vi "qWGI.vi"(0 "System no.":i32=1 min=1 max=4 step=1, 2 "Generator ID":string[](array[string]), 3 "All IDs?":bool, 4 "identifier?":bool=TRUE, 5 "error in":errorcluster) -> (14 "WGI parameter":i32[](array[numeric]), 19 "error out":errorcluster)   [LabVIEW 2026]
doc: "Returns the index of the currently output wave point.\n\nE-709: Generator ID can be 1. If All IDs? = TRUE, then identifier? must be FALSE."
panel:
  # "Returns the index of the currently output wave point"
  # "If all IDs: use"
  # "Query"
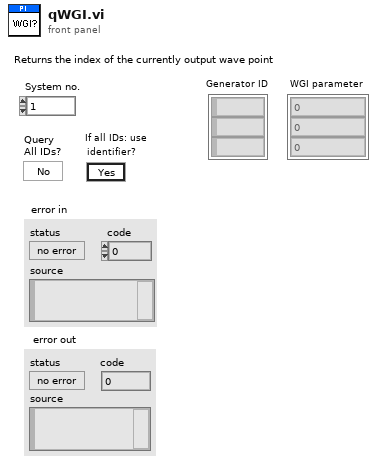
[diagram p1: front panel]
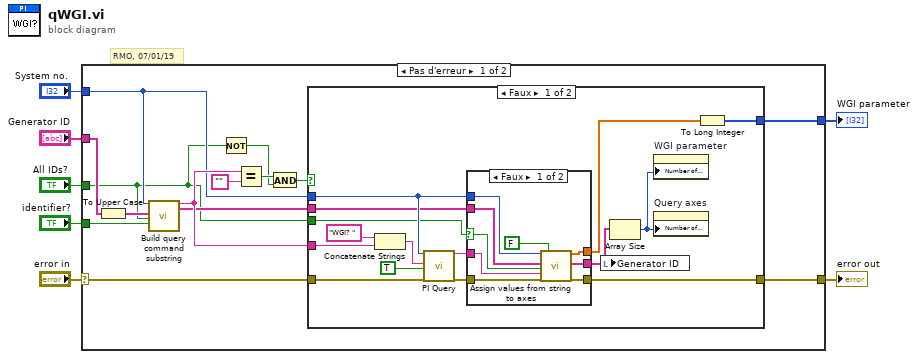
[diagram p0: block diagram]
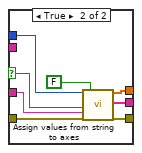
[diagram p2: hidden frame]
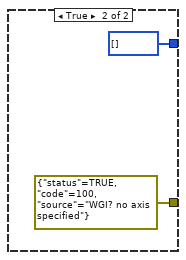
[diagram p3: hidden frame]
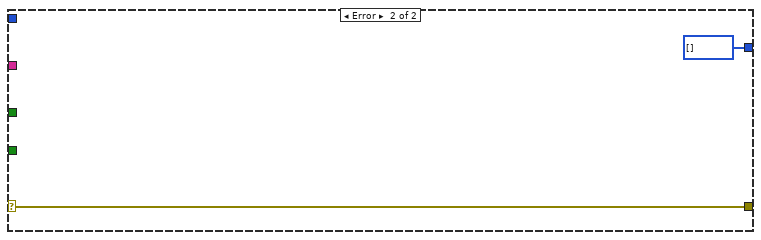
[diagram p4: hidden frame]
diagram:
  # "RMO, 07/01/19"
  n1 = case shown="Pas d'erreur" "error in" {
    selector: "error in" -> [w10 w57]
    tunnel: [w21 i32[] []] -> w7
    tunnel: "Generator ID" -> [w20 _]
    tunnel: [w8 w57] -> w5
    tunnel: "identifier?" -> [w17 _]
    tunnel: "System no." -> [w15 _]
    tunnel: "All IDs?" -> [w11 _]
    frame No Error {
      n2 = To Upper Case(1:w20) -> (0:w18:string[])
      n3 = call "Build query command substring.vi"("System no."=w15, "Axes to query in"=w18, "Query\nAll axes?"=w11, "For all axes: use\nAxis identifier?"=w17) -> ("Command substring"=w16:string, "Axes to query out"=w14:string[])  [unwired: 2 in, 12 out]
      n4 = Not(x=w11) -> (.not. x?=w12:bool)
      n5 = Equal?(x=w16, y="" ("x")) -> (x = y?=w13:bool)
      n6 = And(x=w13, y=w12) -> (x .and. y?=w9:bool)
      n7 = case shown="Faux" w9 {
        tunnel: [w22 i32[] []] -> w21
        tunnel: w16 -> [w33 _]
        tunnel: w15 -> [w32 _]
        tunnel: w14 -> [w31 _]
        tunnel: w11 -> [w30 _]
        tunnel: w10 -> [w27 _]
        tunnel: [w26 errorcluster {"status"=TRUE, "code"=100, "source"="WGI? no axis specified"} ("error out")] -> w8
        frame False {
          n8 = Concatenate Strings("WGI? ", w33) -> (w34:string)
          n9 = call "PI Query.vi"("System no."=w32, "String to send"=w34, "Attach termination char.?"=TRUE ("Attach Linefeed?"), "error in"=w27) -> ("String read"=w24:string, "error out"=w25:errorcluster)  [unwired: 3 in, 11 out]
          n10 = case shown="Faux" w30 {
            selector: w30 -> [w39 w49]
            tunnel: [w45 w48] -> w23
            tunnel: w32 -> [w44 w53]
            tunnel: w31 -> [w43 _]
            tunnel: w24 -> [w42 w52]
            tunnel: [w41 w51] -> w26
            tunnel: w25 -> [w40 w50]
            tunnel: [w38 w47] -> w28
            frame False {
              n11 = call "Assign values from string to axes.vi"("System no."=w44, "Queried axes"=w43, "All axes queried?"=w39, "Input String"=w42, "error in"=w40, "Axes related?"=FALSE) -> ("Values"=w45:dbl[], "Queried axes out"=w38:string[], "error out"=w41:errorcluster)  [unwired: 3 in, 8 out]
            }
            frame True {
              n12 = call "Assign values from string to axes.vi"("System no."=w53, "All axes queried?"=w49, "Input String"=w52, "error in"=w50, "Axes related?"=FALSE) -> ("Values"=w48:dbl[], "Queried axes out"=w47:string[], "error out"=w51:errorcluster)  [unwired: 4 in, 8 out]
            }
          }
          n13 = local write "Generator ID"(w28) -> ()
          n14 = Array Size(array=w28) -> (size(s)=w29:i32)
          n15 = property on="WGI parameter" class="Tabl (strict)"("Number of Rows"=w29) -> ()  [unwired: 2 in, 2 out]
          n16 = property on="Query axes" class="Tabl (strict)"("Number of Rows"=w29) -> ()  [unwired: 2 in, 2 out]
          n17 = To Long Integer(number=w23) -> (32bit integer=w22:i32[])
        }
        frame True {
        }
      }
    }
    frame Error {
    }
  }
  "error out" <- w5
  "WGI parameter" <- w7
